vi "HandleCmd.vi"(8 "error in (no error)":errorcluster, 11 "NeedleValve in":refnum<class "NeedleValve.lvclass">) -> (0 "error out":errorcluster, 3 "NeedleValve out":refnum<class "NeedleValve.lvclass">)   [LabVIEW 2019, in "NeedleValve.lvclass"]
uses:
  NeedleValve.lvclass
  D:/GIT H4000/H4000/src/Device_class/Device.lvclass
  Device_class/Device.lvclass/Device.ctl
  NeedleValve.lvclass/NeedleValve.ctl
  Proccess_class/Proccess.lvclass/Proccess.ctl
  modbus engine custom/MB_ENGINE_class/cmd enum.ctl
  TypeDef/Needle Valve State.ctl
  a659752c-c270-45de-af0a-8377def0b31c.vi
  70b31653-b39a-4d19-a66b-143deb4fa3eb.vi
  Proccess_class/GetNames.vi
  Proccess_class/GetLogger.vi
  Device_class/Device.lvclass
  D:/GIT H4000/H4000/src/Proccess_class/Proccess.lvclass
  Logger_class/WriteEvent.vi
  <vilib>/addons/_JKI.lib/Serialization/JSON/Library/Unflatten From JSON String.vi
  MessageInterface_class/MessageInterface.lvclass
  modbus engine custom/MB_ENGINE_class/MB_ENGINE.lvclass
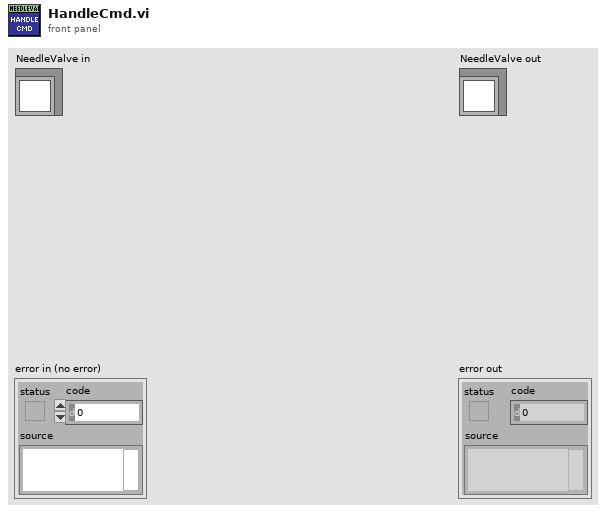
[diagram p1: front panel]
types:
  T1 = typedef "MessageInterface.lvclass/Message.ctl" = cluster{"name":string, "value":string, "receiver host":string, "receiver process":string, "source host":string, "source process":string}
  T2 = typedef "Needle Valve State.ctl" = enum16{"STOPED", "CLOSED", "OPENED", "OPENING", "CLOSING", "FULL_CLOSE", "PREP_OPEN"}
  T3 = typedef "Needle Valve Data.ctl" = cluster{"Engine State":T4, "StateValveModbus":T2, "Alarms":T5, "RAW":i32, "Angele":dbl, "Step":i32, "Encoder":i32, "Kinematic":T6, "Limits":T7, "EncoderMax":i32, "Counter Max Dont Update":i32, "EncoderMin":i32, "Counter Min Dont Update":i32, "Prepere Counter":i32, "STEP INIT":i32, "offset - Angel":dbl}
  T4 = typedef "MB_ENGINE.lvclass/Engine State.ctl" = u16
  T5 = typedef "MB_ENGINE.lvclass/Engine Alarms.ctl" = cluster{"OL":bool, "TF":bool, "STL":bool, "OCP":bool, "CPUV":bool, "UVLO":bool, "SPI_ERROR":bool, "Fault":bool, "OL 2":bool, "TF 2":bool, "STL 2":bool, "OCP 2":bool, "CPUV 2":bool, "UVLO 2":bool, "reserved":bool, "InitDone":bool}
  T6 = typedef "MB_ENGINE.lvclass/Settings.ctl" = cluster{"ACC Steps Per Sec^2":u16, "DEC Steps Per Sec^2":u16, "Min Velosity Step Per Sec":u16, "Max Velosity Step Per Sec":u16, "MicroStep":u16}
  T7 = typedef "MB_ENGINE.lvclass/Limits Status.ctl" = cluster{"Fault 2 Switch":bool, "Fault 1 Switch":bool, "Center(Home)":bool, "Lower Limit":bool, "Upper Limit":bool}
  T8 = typedef "MB_ENGINE.lvclass/cmd enum.ctl" = u16
  T9 = typedef "Needle Valve Settings.ctl" = cluster{"average size":i32, "open force":u16, "close force":u16, "open settings":T6, "close settings":T6, "Offset angle":dbl, "Start angle":dbl}
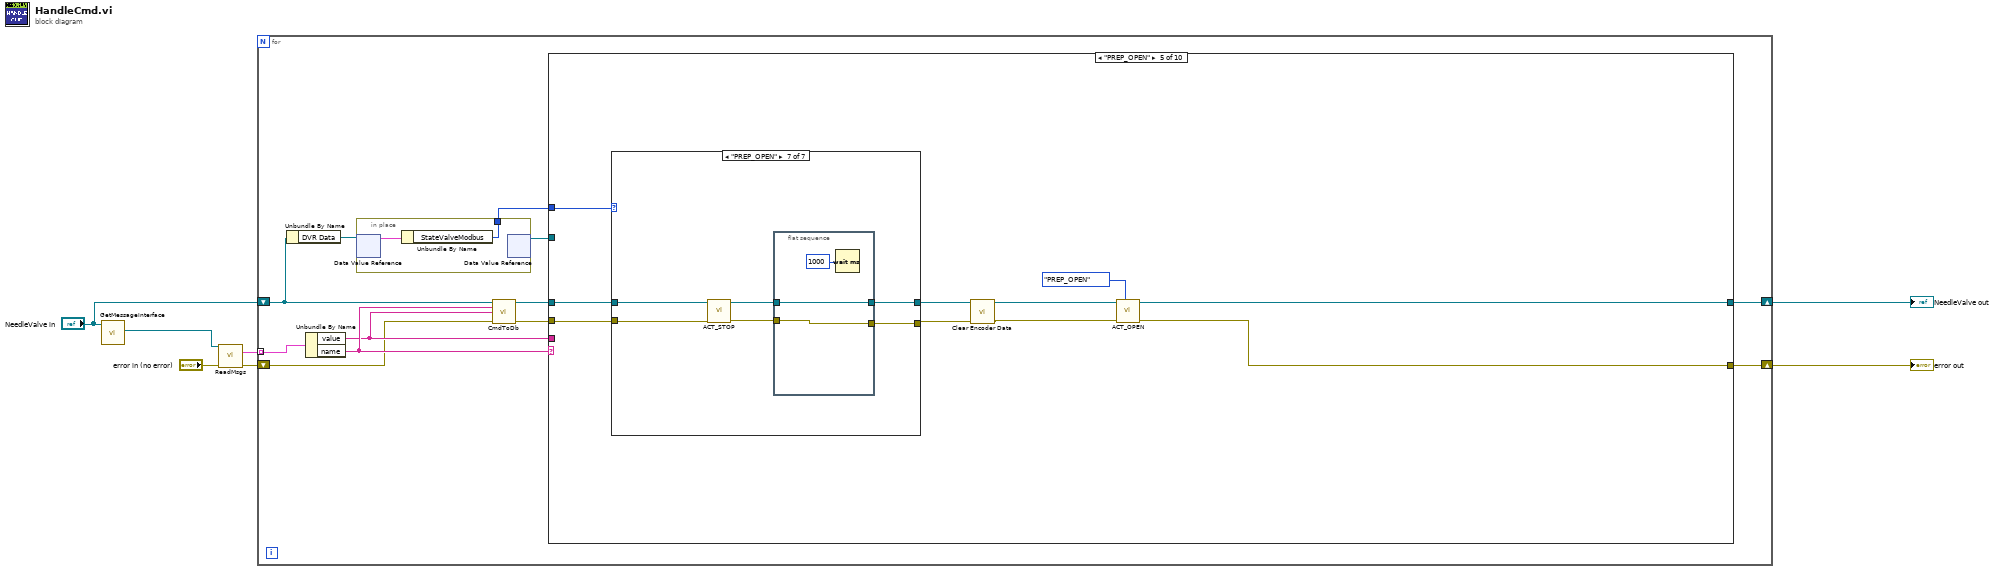
[diagram p0: block diagram]
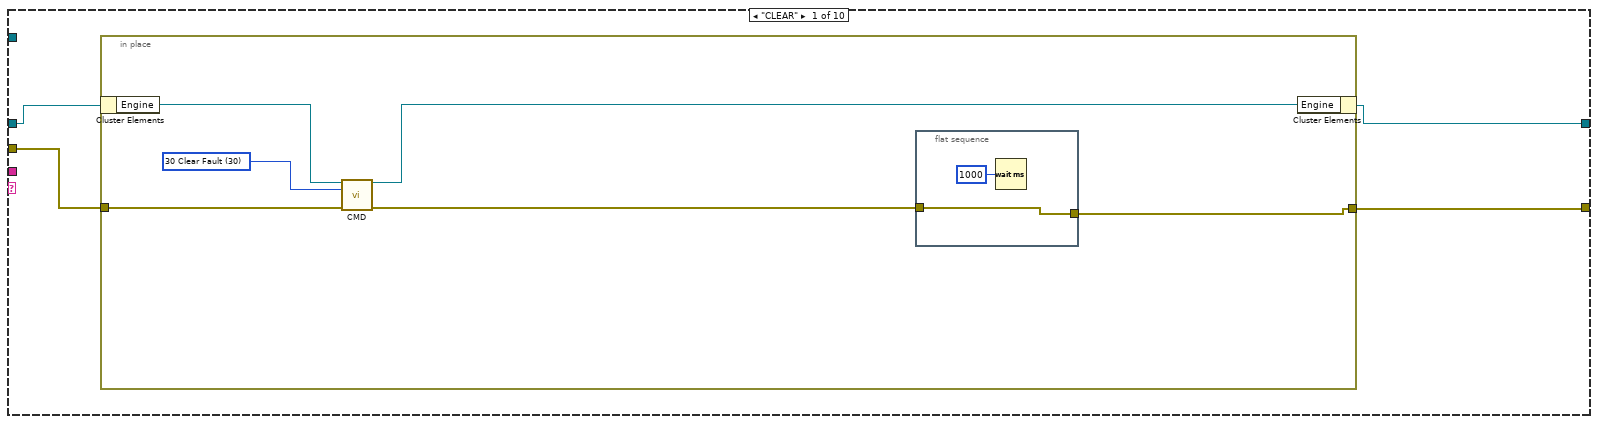
[diagram p2: hidden frame]
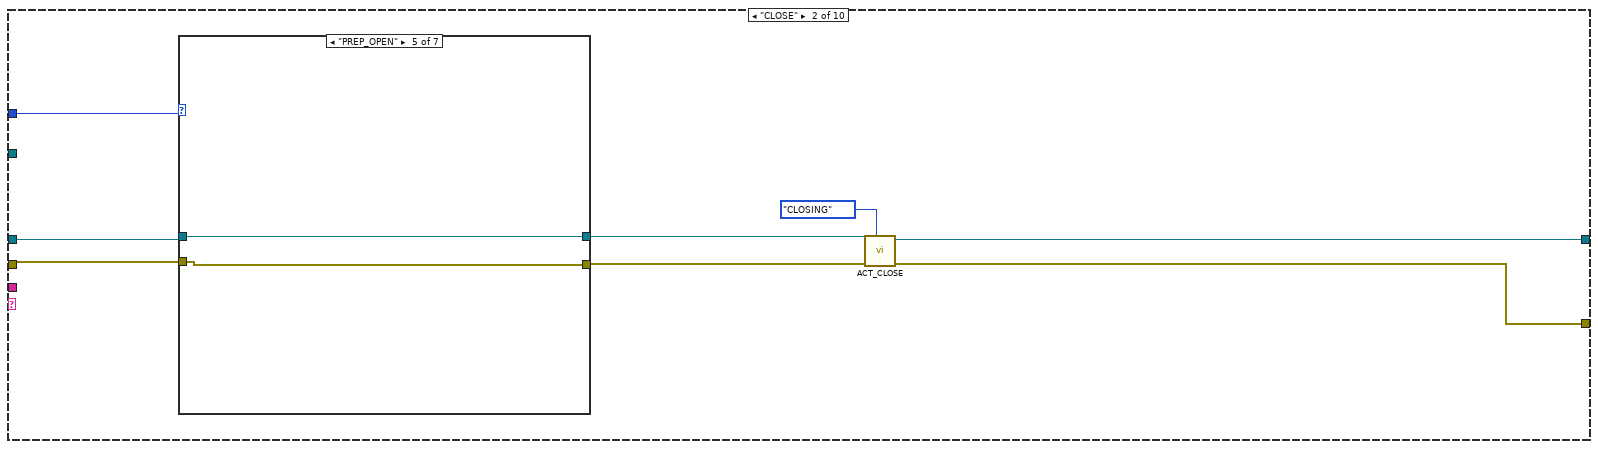
[diagram p3: hidden frame]
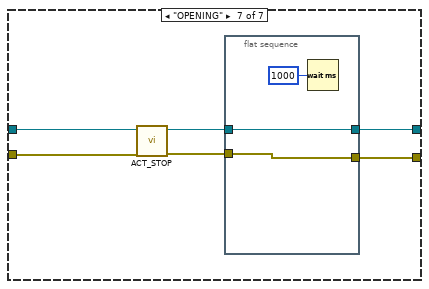
[diagram p9: hidden frame]
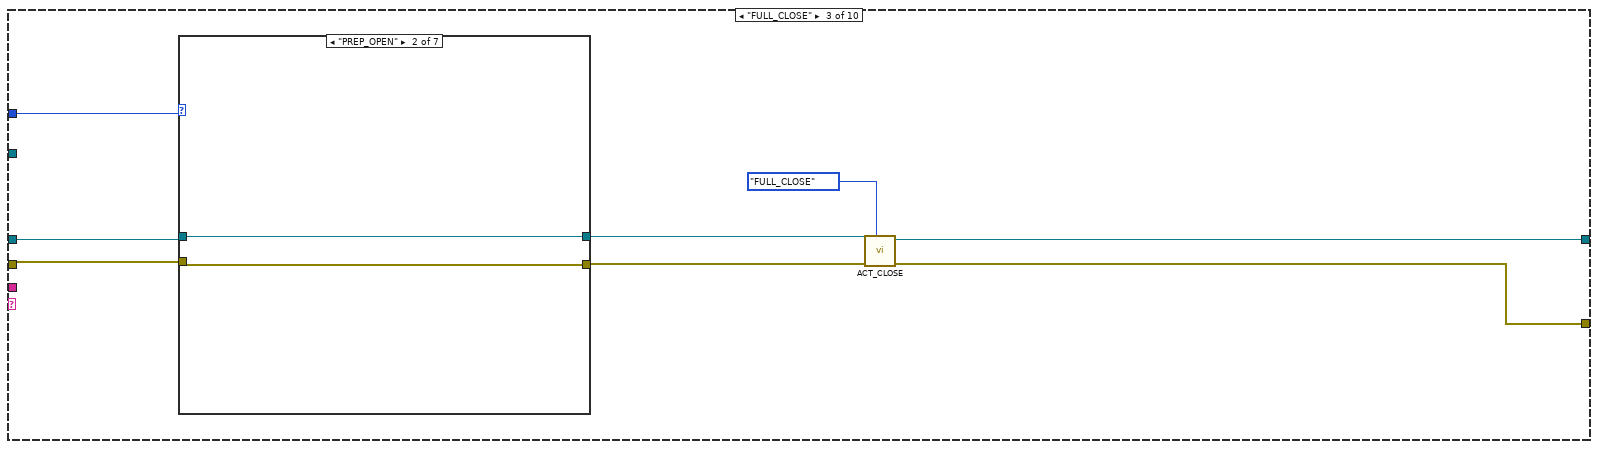
[diagram p10: hidden frame]
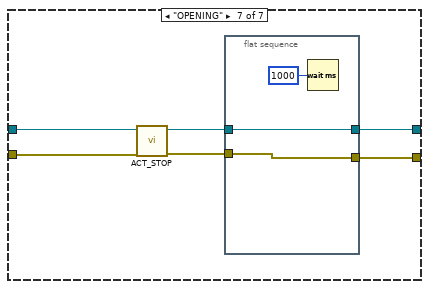
[diagram p16: hidden frame]
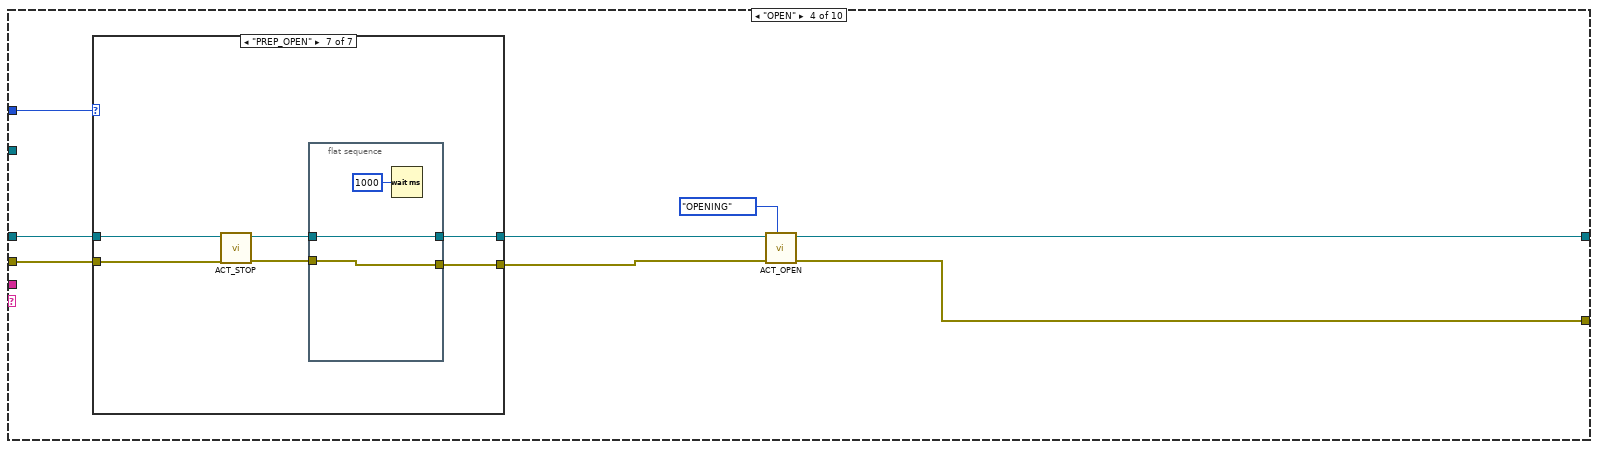
[diagram p17: hidden frame]
diagram:
  n1 = call "GetMessageInterface.vi"("Device in"="NeedleValve in") -> ("MessageInterface"=w7:refnum<class "MessageInterface.lvclass">)  [unwired: 10 in]
  n2 = call-dynamic "ReadMsgs.vi"("reference in"=w7, "error in (no error)"="error in (no error)") -> ("msgs"=w5:T1[], "error out"=w6:errorcluster)  [unwired: 11 in, 1 out]
  n3 = for {
    shift-right: [w18] -> w1
    shift-left: w6 -> [w14]
    tunnel: w5 -> [w19] mode=indexing
    shift-right: [w17] -> w2
    shift-left: "NeedleValve in" -> [w11]
    n4 = Unbundle By Name(w11) -> ("DVR Data"=w10:refnum<data-value>)
    n5 = Unbundle By Name(w19) -> ("value"=w15:string, "name"=w16:string)
    n6 = in-place {
      in-place-border: [w20] -> w9
      n7 = in-place-dvr #1(w10) -> (w21:T3)  [unwired: 1 out]
      n8 = Unbundle By Name(w21) -> ("StateValveModbus"=w20:T2)
      n9 = in-place-dvr #1() -> (w8:refnum<data-value>)  [unwired: 1 in, 1 out]
    }
    n10 = call "CmdToDb.vi"("reference in"=w11, "CMD"=w16, "Value"=w15, "error in (no error)"=w14) -> ("reference out"=w12:refnum<class "NeedleValve.lvclass">, "error out"=w13:errorcluster)  [unwired: 10 in]
    n11 = case shown="\"PREP_OPEN\"" w16 {
      tunnel: w12 -> [w25 w39 w68 w95 w134 w170 w184 w191 w199 w205]
      tunnel: [w22 w40 w69 w98 w136 w167 w180 w193 w198 w205] -> w17
      tunnel: [w23 w41 w70 w99 w137 w168 w179 w192 w196 w204] -> w18
      tunnel: w13 -> [w24 w38 w67 w93 w133 w169 w185 w194 w197 w204]
      tunnel: w15 -> [_ _ _ _ _ w166 w183 _ _ _]
      tunnel: w9 -> [_ w35 w64 w97 w135 _ _ _ _ _]
      tunnel: w8 -> [_ _ _ _ _ _ _ _ w195 _]
      frame "CLEAR" {
        n12 = in-place {
          in-place-border: w24 -> [w31]
          in-place-border: [w27] -> w23
          w29 = T8 30 items=["0 Idle"=0, "1 GoTo Absolute Position"=1, "2 GoTo Relative"=2, "10 GoTo Home Position"=10, "11 Set Home Position"=11, "12 Set FindHome Mode"=12, "13 Reset FindHome Mode"=13, "14 Get FindHome State"=14, "20 Hard Stop"=20, "21 HiZ Stop"=21, "22 Soft Stop"=22, "30 Clear Fault"=30, "40 Encoder Set Home"=40, "70 Driver Init"=70] ("cmd to write")
          n13 = in-place-cluster #2(w25) -> ("Engine"=w30:refnum<class "MB_ENGINE.lvclass">)
          n14 = call "CMD.vi"("class data in"=w30, "cmd to write"=w29, "error in (no error)"=w31) -> ("class data out"=w28:refnum<class "MB_ENGINE.lvclass">, "error out"=w26:errorcluster)  [unwired: 11 in]
          n15 = flat-sequence {
            tunnel: [w32] -> w27
            tunnel: w26 -> [w32]
            frame #0 {
              n16 = Wait (ms)(milliseconds to wait=u32 1000) -> ()  [unwired: 1 out]
            }
          }
          n17 = in-place-cluster #2("Engine"=w28) -> (w22:refnum<class "NeedleValve.lvclass">)
        }
      }
      frame "CLOSE" {
        n18 = case shown="\"PREP_OPEN\"" w35 {
          tunnel: [w43 w45 w47 w49 w51 w53 w55] -> w37
          tunnel: w39 -> [w43 w45 w47 w49 w51 w53 w59]
          tunnel: [w42 w44 w46 w48 w50 w52 w57] -> w36
          tunnel: w38 -> [w42 w44 w46 w48 w50 w52 w58]
          frame "STOPED" {
          }
          frame "FULL_CLOSE" {
          }
          frame "CLOSED" {
          }
          frame "OPENED" {
          }
          frame "PREP_OPEN" {
          }
          frame "CLOSING" {
          }
          frame "OPENING" {
            n19 = call "ACT_STOP.vi"("error in (no error)"=w58, "NeedleValve in"=w59) -> ("error out"=w56:errorcluster, "NeedleValve out"=w54:refnum<class "NeedleValve.lvclass">)  [unwired: 8 in]
            n20 = flat-sequence {
              tunnel: [w62] -> w57
              tunnel: w56 -> [w62]
              tunnel: [w61] -> w55
              tunnel: w54 -> [w61]
              frame #0 {
                n21 = Wait (ms)(milliseconds to wait=u32 1000) -> ()  [unwired: 1 out]
              }
            }
          }
        }
        n22 = call "ACT_CLOSE.vi"("StateValveModbus"=Needle_Valve_State."CLOSING", "error in (no error)"=w36, "NeedleValve in"=w37) -> ("error out"=w41:errorcluster, "NeedleValve out"=w40:refnum<class "NeedleValve.lvclass">)  [unwired: 7 in]
      }
      frame "FULL_CLOSE" {
        n23 = case shown="\"PREP_OPEN\"" w64 {
          tunnel: [w72 w74 w76 w78 w80 w82 w84] -> w66
          tunnel: w68 -> [w72 w74 w76 w78 w80 w82 w88]
          tunnel: [w71 w73 w75 w77 w79 w81 w86] -> w65
          tunnel: w67 -> [w71 w73 w75 w77 w79 w81 w87]
          frame "STOPED" {
          }
          frame "PREP_OPEN" {
          }
          frame "FULL_CLOSE" {
          }
          frame "CLOSED" {
          }
          frame "OPENED" {
          }
          frame "CLOSING" {
          }
          frame "OPENING" {
            n24 = call "ACT_STOP.vi"("error in (no error)"=w87, "NeedleValve in"=w88) -> ("error out"=w85:errorcluster, "NeedleValve out"=w83:refnum<class "NeedleValve.lvclass">)  [unwired: 8 in]
            n25 = flat-sequence {
              tunnel: [w91] -> w86
              tunnel: w85 -> [w91]
              tunnel: [w90] -> w84
              tunnel: w83 -> [w90]
              frame #0 {
                n26 = Wait (ms)(milliseconds to wait=u32 1000) -> ()  [unwired: 1 out]
              }
            }
          }
        }
        n27 = call "ACT_CLOSE.vi"("StateValveModbus"=Needle_Valve_State."FULL_CLOSE", "error in (no error)"=w65, "NeedleValve in"=w66) -> ("error out"=w70:errorcluster, "NeedleValve out"=w69:refnum<class "NeedleValve.lvclass">)  [unwired: 7 in]
      }
      frame "OPEN" {
        n28 = case shown="\"PREP_OPEN\"" w97 {
          tunnel: [w101 w103 w105 w107 w109 w111 w120] -> w96
          tunnel: w95 -> [w101 w103 w105 w107 w109 w115 w124]
          tunnel: [w100 w102 w104 w106 w108 w113 w122] -> w94
          tunnel: w93 -> [w100 w102 w104 w106 w108 w114 w123]
          frame "STOPED" {
          }
          frame "CLOSED" {
          }
          frame "FULL_CLOSE" {
          }
          frame "OPENED" {
          }
          frame "OPENING" {
          }
          frame "CLOSING" {
            n29 = call "ACT_STOP.vi"("error in (no error)"=w114, "NeedleValve in"=w115) -> ("error out"=w112:errorcluster, "NeedleValve out"=w110:refnum<class "NeedleValve.lvclass">)  [unwired: 8 in]
            n30 = flat-sequence {
              tunnel: [w118] -> w113
              tunnel: w112 -> [w118]
              tunnel: [w117] -> w111
              tunnel: w110 -> [w117]
              frame #0 {
                n31 = Wait (ms)(milliseconds to wait=u32 1000) -> ()  [unwired: 1 out]
              }
            }
          }
          frame "PREP_OPEN" {
            n32 = call "ACT_STOP.vi"("error in (no error)"=w123, "NeedleValve in"=w124) -> ("error out"=w121:errorcluster, "NeedleValve out"=w119:refnum<class "NeedleValve.lvclass">)  [unwired: 8 in]
            n33 = flat-sequence {
              tunnel: [w127] -> w122
              tunnel: w121 -> [w127]
              tunnel: [w126] -> w120
              tunnel: w119 -> [w126]
              frame #0 {
                n34 = Wait (ms)(milliseconds to wait=u32 1000) -> ()  [unwired: 1 out]
              }
            }
          }
        }
        n35 = call "ACT_OPEN.vi"("Needle Valve Data.StateValveModbus"=Needle_Valve_State."OPENING", "error in (no error)"=w94, "NeedleValve in"=w96) -> ("error out"=w99:errorcluster, "NeedleValve out"=w98:refnum<class "NeedleValve.lvclass">)  [unwired: 7 in]
      }
      frame "PREP_OPEN" {
        n36 = case shown="\"PREP_OPEN\"" w135 {
          tunnel: [w139 w141 w143 w145 w147 w149 w158] -> w131
          tunnel: w134 -> [w139 w141 w143 w145 w147 w153 w162]
          tunnel: [w138 w140 w142 w144 w146 w151 w160] -> w130
          tunnel: w133 -> [w138 w140 w142 w144 w146 w152 w161]
          frame "STOPED" {
          }
          frame "CLOSED" {
          }
          frame "FULL_CLOSE" {
          }
          frame "OPENED" {
          }
          frame "OPENING" {
          }
          frame "CLOSING" {
            n37 = call "ACT_STOP.vi"("error in (no error)"=w152, "NeedleValve in"=w153) -> ("error out"=w150:errorcluster, "NeedleValve out"=w148:refnum<class "NeedleValve.lvclass">)  [unwired: 8 in]
            n38 = flat-sequence {
              tunnel: [w156] -> w151
              tunnel: w150 -> [w156]
              tunnel: [w155] -> w149
              tunnel: w148 -> [w155]
              frame #0 {
                n39 = Wait (ms)(milliseconds to wait=u32 1000) -> ()  [unwired: 1 out]
              }
            }
          }
          frame "PREP_OPEN" {
            n40 = call "ACT_STOP.vi"("error in (no error)"=w161, "NeedleValve in"=w162) -> ("error out"=w159:errorcluster, "NeedleValve out"=w157:refnum<class "NeedleValve.lvclass">)  [unwired: 8 in]
            n41 = flat-sequence {
              tunnel: [w165] -> w160
              tunnel: w159 -> [w165]
              tunnel: [w164] -> w158
              tunnel: w157 -> [w164]
              frame #0 {
                n42 = Wait (ms)(milliseconds to wait=u32 1000) -> ()  [unwired: 1 out]
              }
            }
          }
        }
        n43 = call "Clear Encoder Data.vi"("reference in"=w131, "error in (no error)"=w130) -> ("reference out"=w129:refnum<class "NeedleValve.lvclass">, "error out"=w128:errorcluster)  [unwired: 12 in]
        n44 = call "ACT_OPEN.vi"("Needle Valve Data.StateValveModbus"=Needle_Valve_State."PREP_OPEN", "error in (no error)"=w128, "NeedleValve in"=w129) -> ("error out"=w137:errorcluster, "NeedleValve out"=w136:refnum<class "NeedleValve.lvclass">)  [unwired: 7 in]
      }
      frame "SET_CMD" {
        n45 = in-place {
          in-place-border: w169 -> [w175]
          in-place-border: [w176] -> w168
          in-place-border: w166 -> [w174]
          w173 = T8 0 items=["0 Idle"=0, "1 GoTo Absolute Position"=1, "2 GoTo Relative"=2, "10 GoTo Home Position"=10, "11 Set Home Position"=11, "12 Set FindHome Mode"=12, "13 Reset FindHome Mode"=13, "14 Get FindHome State"=14, "20 Hard Stop"=20, "21 HiZ Stop"=21, "22 Soft Stop"=22, "30 Clear Fault"=30, "40 Encoder Set Home"=40, "70 Driver Init"=70] ("cmd to write")
          n46 = in-place-cluster #3(w170) -> ("Engine"=w178:refnum<class "MB_ENGINE.lvclass">)
          n47 = call "ConvertMsgToVariant.vim"("Type and Defaults"=w173, "Value"=w174, "error in (no error)"=w175) -> ("data"=w172:T8, "error out"=w171:errorcluster)  [unwired: 11 in]
          n48 = call "CMD.vi"("class data in"=w178, "cmd to write"=w172, "error in (no error)"=w171) -> ("class data out"=w177:refnum<class "MB_ENGINE.lvclass">, "error out"=w176:errorcluster)  [unwired: 11 in]
          n49 = in-place-cluster #3("Engine"=w177) -> (w167:refnum<class "NeedleValve.lvclass">)
        }
      }
      frame "SET_SETTINGS" {
        n50 = in-place {
          in-place-border: w185 -> [w190]
          in-place-border: w183 -> [w188]
          in-place-border: [w187] -> w182
          n51 = in-place-cluster #4(w184) -> ("Needle Valve Settings"=w189:T9)
          n52 = call "ConvertMsgToVariant.vim"("Type and Defaults"=w189, "Value"=w188, "error in (no error)"=w190) -> ("data"=w186:T9, "error out"=w187:errorcluster)  [unwired: 11 in]
          n53 = in-place-cluster #4("Needle Valve Settings"=w186) -> (w181:refnum<class "NeedleValve.lvclass">)
        }
        n54 = call-dynamic "WriteConfig.vi"("reference in"=w181, "error in (no error)"=w182) -> ("reference out"=w180:refnum<class "NeedleValve.lvclass">, "error out"=w179:errorcluster)  [unwired: 12 in]
      }
      frame "SET_OFFSET" {
        n55 = call "Set Offset.vi"("error in (no error)"=w194, "NeedleValve in"=w191) -> ("error out"=w192:errorcluster, "NeedleValve out"=w193:refnum<class "NeedleValve.lvclass">)  [unwired: 8 in]
      }
      frame "STOP" {
        n56 = in-place {
          in-place-border: [w200] -> _
          n57 = in-place-dvr #5(w195) -> (w203:T3, w200:errorcluster)
          n58 = Bundle By Name(cluster=w203, "StateValveModbus"=Needle_Valve_State."STOPED" ("Needle Valve Data.StateValveModbus")) -> (w202:T3)
          n59 = in-place-dvr #5(w202) -> ()  [unwired: 2 out]
        }
        n60 = call "ACT_STOP.vi"("error in (no error)"=w197, "NeedleValve in"=w199) -> ("error out"=w196:errorcluster, "NeedleValve out"=w198:refnum<class "NeedleValve.lvclass">)  [unwired: 8 in]
      }
      frame Default {
      }
    }
  }
  "error out" <- w1
  "NeedleValve out" <- w2
